vi "Get Self Alias.vi"(7 "jettl in":refnum<class "jettl.lvclass">, 10 "Addresses DVR":refnum<data-value>) -> (2 "Self Alias":string, 5 "jettl out":refnum<class "jettl.lvclass">)   [LabVIEW 2021, in "jettl.lvlib" / "Addresses.lvlib" / "Addresses.lvclass"]
uses:
  Addresses.lvclass
  jettl/jettl.lvclass
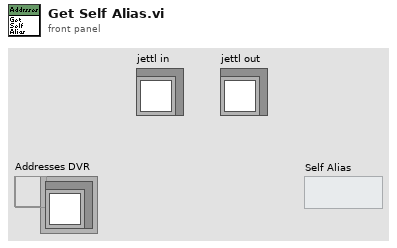
[diagram p1: front panel]
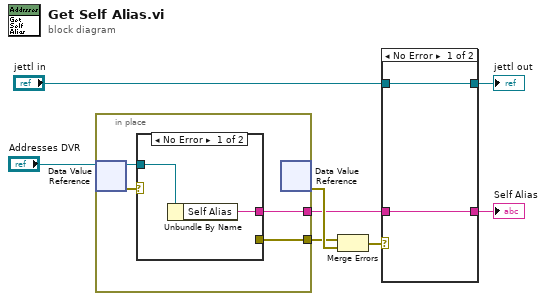
[diagram p0: block diagram]
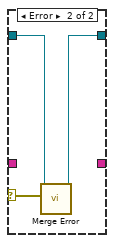
[diagram p2: hidden frame]
diagram:
  n1 = in-place {
    in-place-border: [w12] -> w7
    in-place-border: [w11] -> w3
    n2 = in-place-dvr #1("Addresses DVR") -> (w9:refnum<class "Addresses.lvclass">, w10:errorcluster)
    n3 = case shown="No Error" w10 {
      selector: w10 -> [_ w15]
      tunnel: w9 -> [w14 _]
      tunnel: [_ w15] -> w12
      tunnel: [w13 _] -> w11
      frame No Error {
        n4 = Unbundle By Name(w14) -> ("Self Alias"=w13:string)
      }
      frame Error {
      }
    }
    n5 = in-place-dvr #1() -> (w8:errorcluster)  [unwired: 1 in, 1 out]
  }
  n6 = Merge Errors(w7, w8) -> (w1:errorcluster)
  n7 = case shown="No Error" w1 {
    selector: w1 -> [_ w18]
    tunnel: w3 -> [w16 _]
    tunnel: "jettl in" -> [w17 w20]
    tunnel: [w17 w19] -> w4
    tunnel: [w16 _] -> w2
    frame No Error {
    }
    frame Error {
      n8 = call-dynamic "Merge Error.vi"("Error"=w18, "Merge Error in"=w20) -> ("Merge Error out"=w19:refnum<class "jettl.lvclass">)  [unwired: 9 in]
    }
  }
  "Self Alias" <- w2
  "jettl out" <- w4
